vi "Init UI XY Graph.vi"(7 "XY Graph Other":refnum<vi>, 8 "Ось Y":i32[](array[numeric]), 9 "Ось Х":i32, 10 "Array Lable":string[](array[string]), 11 "XY Graph Time in ref":refnum<vi>) -> (0 "error out":errorcluster, 3 "XY Graph ref":refnum<vi>)   [LabVIEW 2023, in "Graph_data_collector.lvlib" / "Graph_UI.lvlib"]
uses:
  Graph_UI.lvlib
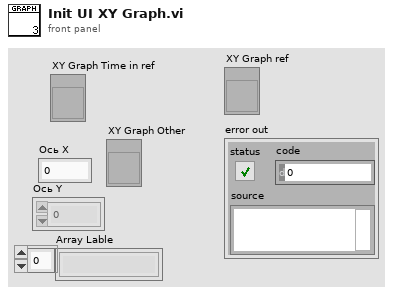
[diagram p1: front panel]
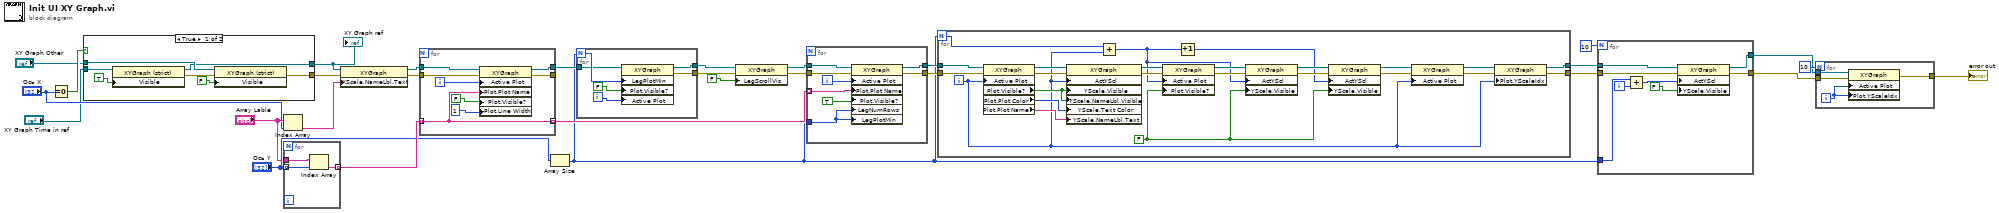
[diagram p0: block diagram]
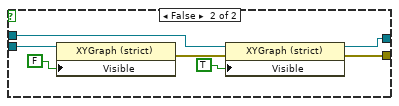
[diagram p2: hidden frame]
diagram:
  n1 = Equal To 0?(x="Ось Х") -> (x = 0?=w8:bool)
  n2 = case shown="True" w8 {
    tunnel: [w36 w43] -> w10
    tunnel: [w30 w42] -> w9
    tunnel: "XY Graph Other" -> [w34 w40]
    tunnel: "XY Graph Time in ref" -> [w31 w37]
    frame True {
      n3 = property on="Property Node" class="XYGraph (strict)"(reference=w31, "Visible"=TRUE) -> (reference out=w30:refnum<vi>, error out=w35:errorcluster)  [unwired: 1 in]
      n4 = property on="Property Node" class="XYGraph (strict)"(reference=w34, error in=w35, "Visible"=FALSE) -> (error out=w36:errorcluster)  [unwired: 1 out]
    }
    frame False {
      n5 = property on="Property Node" class="XYGraph (strict)"(reference=w37, "Visible"=FALSE) -> (error out=w41:errorcluster)  [unwired: 1 in, 1 out]
      n6 = property on="Property Node" class="XYGraph (strict)"(reference=w40, error in=w41, "Visible"=TRUE) -> (reference out=w42:refnum<vi>, error out=w43:errorcluster)
    }
  }
  "XY Graph ref" <- w9
  n7 = Index Array(array="Array Lable", index="Ось Х") -> (element=w21:string)
  n8 = for {
    tunnel: "Array Lable" -> [w46]
    tunnel: "Ось Y" -> [w45] mode=indexing
    tunnel: [w44] -> w22 mode=indexing
    n9 = Index Array(array=w46, index=w45) -> (element=w44:string)
  }
  n10 = property on="Property Node" class="XYGraph"(reference=w9, error in=w10, "XScale.NameLbl.Text"=w21) -> (reference out=w13:refnum<vi>, error out=w12:errorcluster)
  n11 = for {
    tunnel: w22 -> [w50] mode=indexing
    tunnel: w12 -> [w54]
    tunnel: [w53] -> _
    tunnel: [w50] -> w23 mode=indexing
    tunnel: w13 -> [w48]
    tunnel: [w47] -> w29
    i -> [w49]
    n12 = property on="Property Node" class="XYGraph"(reference=w48, error in=w54, "Active Plot"=w49, "Plot.Plot Name"=w50, "Plot.Visible?"=FALSE ("Plot.Visible"), "Plot.Line Width"=u8 1) -> (reference out=w47:refnum<vi>, error out=w53:errorcluster)
  }
  n13 = Array Size(array="Ось Y") -> (size(s)=w15:i32)
  n14 = for {
    N: w15 -> [w60]
    tunnel: [w57] -> w27
    tunnel: [w56] -> w28
    tunnel: w29 -> [w55]
    i -> [w59]
    n15 = property on="Property Node" class="XYGraph"(reference=w55, "LegPlotMin"=w60, "Plot.Visible?"=FALSE ("Plot.Visible"), "Active Plot"=w59) -> (reference out=w56:refnum<vi>, error out=w57:errorcluster)  [unwired: 1 in]
  }
  n16 = property on="Property Node" class="XYGraph"(reference=w28, error in=w27, "LegScrollVis"=FALSE ("Legend:Scrollbar Visible")) -> (reference out=w25:refnum<vi>, error out=w24:errorcluster)
  n17 = for {
    tunnel: w24 -> [w67]
    tunnel: w25 -> [w66]
    tunnel: [w64] -> w19
    tunnel: [w63] -> w20
    tunnel: w23 -> [w62] mode=indexing
    tunnel: w15 -> [w61]
    i -> [w68]
    n18 = property on="Property Node" class="XYGraph"(reference=w66, error in=w67, "Active Plot"=w68, "Plot.Plot Name"=w62, "Plot.Visible?"=TRUE ("Plot.Visible"), "LegNumRows"=w61, "LegPlotMin"=w61) -> (reference out=w63:refnum<vi>, error out=w64:errorcluster)
  }
  n19 = for {
    N: w15 -> [w83]
    tunnel: w19 -> [w92]
    tunnel: w20 -> [w86]
    tunnel: [w69] -> w18
    tunnel: [w70] -> w16
    i -> [w71]
    w77 = FALSE ("Plot.Visible")
    n20 = property on="Property Node" class="XYGraph"(reference=w86, error in=w92, "Active Plot"=w71) -> (reference out=w87:refnum<vi>, error out=w88:errorcluster, "Plot.Visible?"=w90:bool, "Plot.Plot Color"=w89:u32, "Plot.Plot Name"=w91:string)
    n21 = property on="Property Node" class="XYGraph"(reference=w87, error in=w88, "ActYScl"=w71, "YScale.Visible"=w90, "YScale.NameLbl.Visible"=w90, "YScale.Text Color"=w89, "YScale.NameLbl.Text"=w91) -> (reference out=w85:refnum<vi>, error out=w84:errorcluster)
    n22 = Add(x=w83, y=w71) -> (x+y=w78:i32)
    n23 = property on="Property Node" class="XYGraph"(reference=w85, error in=w84, "Active Plot"=w78, "Plot.Visible?"=w77) -> (reference out=w82:refnum<vi>, error out=w81:errorcluster)
    n24 = Increment(x=w78) -> (x+1=w76:i32)
    n25 = property on="Property Node" class="XYGraph"(reference=w82, error in=w81, "ActYScl"=w78, "YScale.Visible"=w77) -> (reference out=w80:refnum<vi>, error out=w79:errorcluster)
    n26 = property on="Property Node" class="XYGraph"(reference=w80, error in=w79, "ActYScl"=w76, "YScale.Visible"=w77) -> (reference out=w75:refnum<vi>, error out=w74:errorcluster)
    n27 = property on="Property Node" class="XYGraph"(reference=w75, error in=w74, "Active Plot"=w71) -> (reference out=w73:refnum<vi>, error out=w72:errorcluster)
    n28 = property on="Property Node" class="XYGraph"(reference=w73, error in=w72, "Plot.YScaleIdx"=w71) -> (reference out=w69:refnum<vi>, error out=w70:errorcluster)
  }
  n29 = for {
    N: 10 -> [_]
    tunnel: w18 -> [w99]
    tunnel: w16 -> [w100]
    tunnel: [w98] -> w3
    tunnel: [w97] -> w1
    tunnel: w15 -> [w93]
    i -> [w95]
    n30 = Add(x=w93, y=w95) -> (x+y=w94:i32)
    n31 = property on="Property Node" class="XYGraph"(reference=w99, error in=w100, "ActYScl"=w94, "YScale.Visible"=FALSE ("Y Scale.Visible")) -> (reference out=w98:refnum<vi>, error out=w97:errorcluster)
  }
  n32 = for {
    N: 10 -> [_]
    tunnel: w3 -> [w104]
    tunnel: [w102] -> w2
    tunnel: w1 -> [w101]
    i -> [w103]
    n33 = property on="Property Node" class="XYGraph"(reference=w104, error in=w101, "Active Plot"=w103, "Plot.YScaleIdx"=w103) -> (error out=w102:errorcluster)  [unwired: 1 out]
  }
  "error out" <- w2
